vi "month.vi"() -> (1 "date":string, 3 "Month Chr":string)   [LabVIEW 2015]
panel:
  out "year":string
  out "day":string
  out "date/time string":string
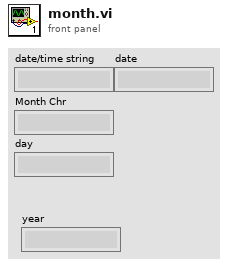
[diagram p1: front panel]
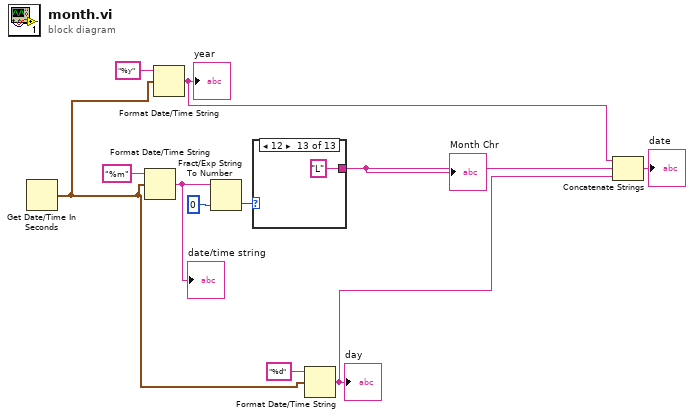
[diagram p0: block diagram]
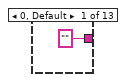
[diagram p2: hidden frame]
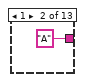
[diagram p3: hidden frame]
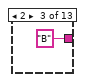
[diagram p4: hidden frame]
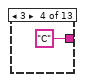
[diagram p5: hidden frame]
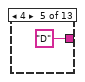
[diagram p6: hidden frame]
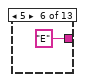
[diagram p7: hidden frame]
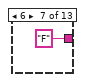
[diagram p8: hidden frame]
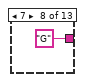
[diagram p9: hidden frame]
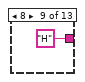
[diagram p10: hidden frame]
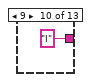
[diagram p11: hidden frame]
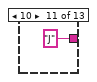
[diagram p12: hidden frame]
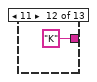
[diagram p13: hidden frame]
diagram:
  n1 = Get Date/Time In Seconds() -> (seconds since 1Jan1904=w1:timestamp)
  n2 = Format Date/Time String(time format string (%c)="%m", seconds (now)=w1) -> (date/time string=w9:string)  [unwired: 1 in]
  "date/time string" <- w9
  n3 = Format Date/Time String(time format string (%c)="%y", seconds (now)=w1) -> (date/time string=w5:string)  [unwired: 1 in]
  "year" <- w5
  n4 = Fract/Exp String To Number(string=w9, default (0 dbl)=0) -> (number=w8:i32)  [unwired: 2 in, 1 out]
  n5 = case shown="12" w8 {
    tunnel: ["" "A" "B" "C" "D" "E" "F" "G" "H" "I" "J" "K" "L"] -> w4
    frame 0, Default {
    }
    frame 1 {
    }
    frame 2 {
    }
    frame 3 {
    }
    frame 4 {
    }
    frame 5 {
    }
    frame 6 {
    }
    frame 7 {
    }
    frame 8 {
    }
    frame 9 {
    }
    frame 10 {
    }
    frame 11 {
    }
    frame 12 {
    }
  }
  "Month Chr" <- w4
  n6 = Format Date/Time String(time format string (%c)="%d", seconds (now)=w1) -> (date/time string=w3:string)  [unwired: 1 in]
  "day" <- w3
  n7 = Concatenate Strings(w5, w4, w3) -> (→"date":string)
